vi "SEScontrol.vi"() -> ()   [LabVIEW 2015]
uses:
  <userlib>/caLab/Private/Get_PV-1D.vi
  user32.dll
  <vilib>/picture/picture.llb/imagedata.ctl
panel:
  out "error out":errorcluster
  out "Waveform Chart":u8(graph)
  out "SES:ScreenCount":u8
  out "SES:Screen":picture
  out "SPEAR_STATE_bool":bool
  out "SPEAR_STATE":dbl
  out "SES:BUSY":bool
  out "SES:Stop_REQ":i8
  out "SES:Run_REQ":i8
  out "SES:Cal_OFF_REQ":i8
  out "SES:Cal_On_REQ":i8
  in  "SES:Cal_Off":bool caption="Play"
  in  "SES:Cal_On":bool caption="Play"
  in  "SES:Kin_Energy":dbl=350.0 min=5.0 max=900.0
  in  "exit":bool
  in  "SES:Run":bool caption="Play"
  in  "SES:Stop":bool
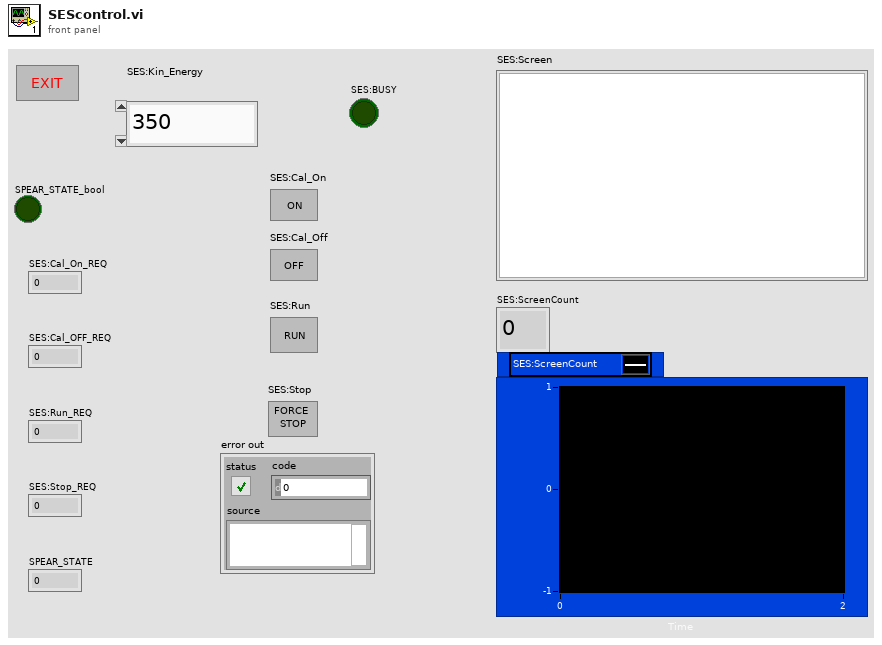
[diagram p1: front panel]
types:
  T1 = typedef "imagedata.ctl" = cluster{"image type":i32, "image depth":i32, "image":u8[], "mask":u8[], "colors":u32[], "Rectangle":cluster{"left":i16, "top":i16, "right":i16, "bottom":i16}}
  T2 = enum16{"Mouse Left", "Mouse Right", "Break", "Mouse Middle", "Backspace", "Tabulator", "FormFeed", "Return", "Shift", "Control", "Alternate", "Pause", "CapsLock", "Escape", "Space", "Page Up", "Page Down", "End", "Home", "Left", "Up", "Right", "Down", "Select", "Print", "Execute", "Snapshot", "Insert", "Delete", "Help", "0", "1", "2", "3", "4", "5", "6", "7", "8", "9", "A", "B", "C", "D", "E", "F", "G", "H", "I", "J", "K", "L", "M", "N", "O", "P", "Q", "R", "S", "T", "U", "V", "W", "X", "Y", "Z", "Win Left", "Win Right", "Context Menu", "Num 0", "Num 1", "Num 2", "Num 3", "Num 4", "Num 5", "Num 6", "Num 7", "Num 8", "Num 9", "Multiply", "Add", "Separator", "Subtract", "Decimal", "Divide", "F1", "F2", "F3", "F4", "F5", "F6", "F7", "F8", "F9", "F10", "F11", "F12", "F13", "F14", "F15", "F16", "F17", "F18", "F19", "F20", "F21", "F22", "F23", "F24", "NumLock", "Scroll", "Shift Left", "Shift Right", "Control Left", "Control Right", "Alternate Left", "Alternate Right", "Attn", "CrSel", "ExSel", "ErEOF", "Play", "Zoom", "Noname", "PA1", "OEM Clear", "Germany <", "Germany ^", "Germany ß", "Germany ´", "Germany ü", "Germany +", "Germany ö", "Germany ä", "Germany #", "Germany ,", "Germany .", "Germany -"}
  T3 = enum16{"NO", "SHIFT", "CTRL", "ALT", "SHIFT + CTRL", "SHIFT + ALT", "CTRL + ALT", "SHIFT + CTRL + ALT"}
  T4 = typedef "LVRectTypeDef.ctl" = cluster{"left":i16, "top":i16, "right":i16, "bottom":i16}
  T5 = typedef "WindowHandle" = refnum<k1>
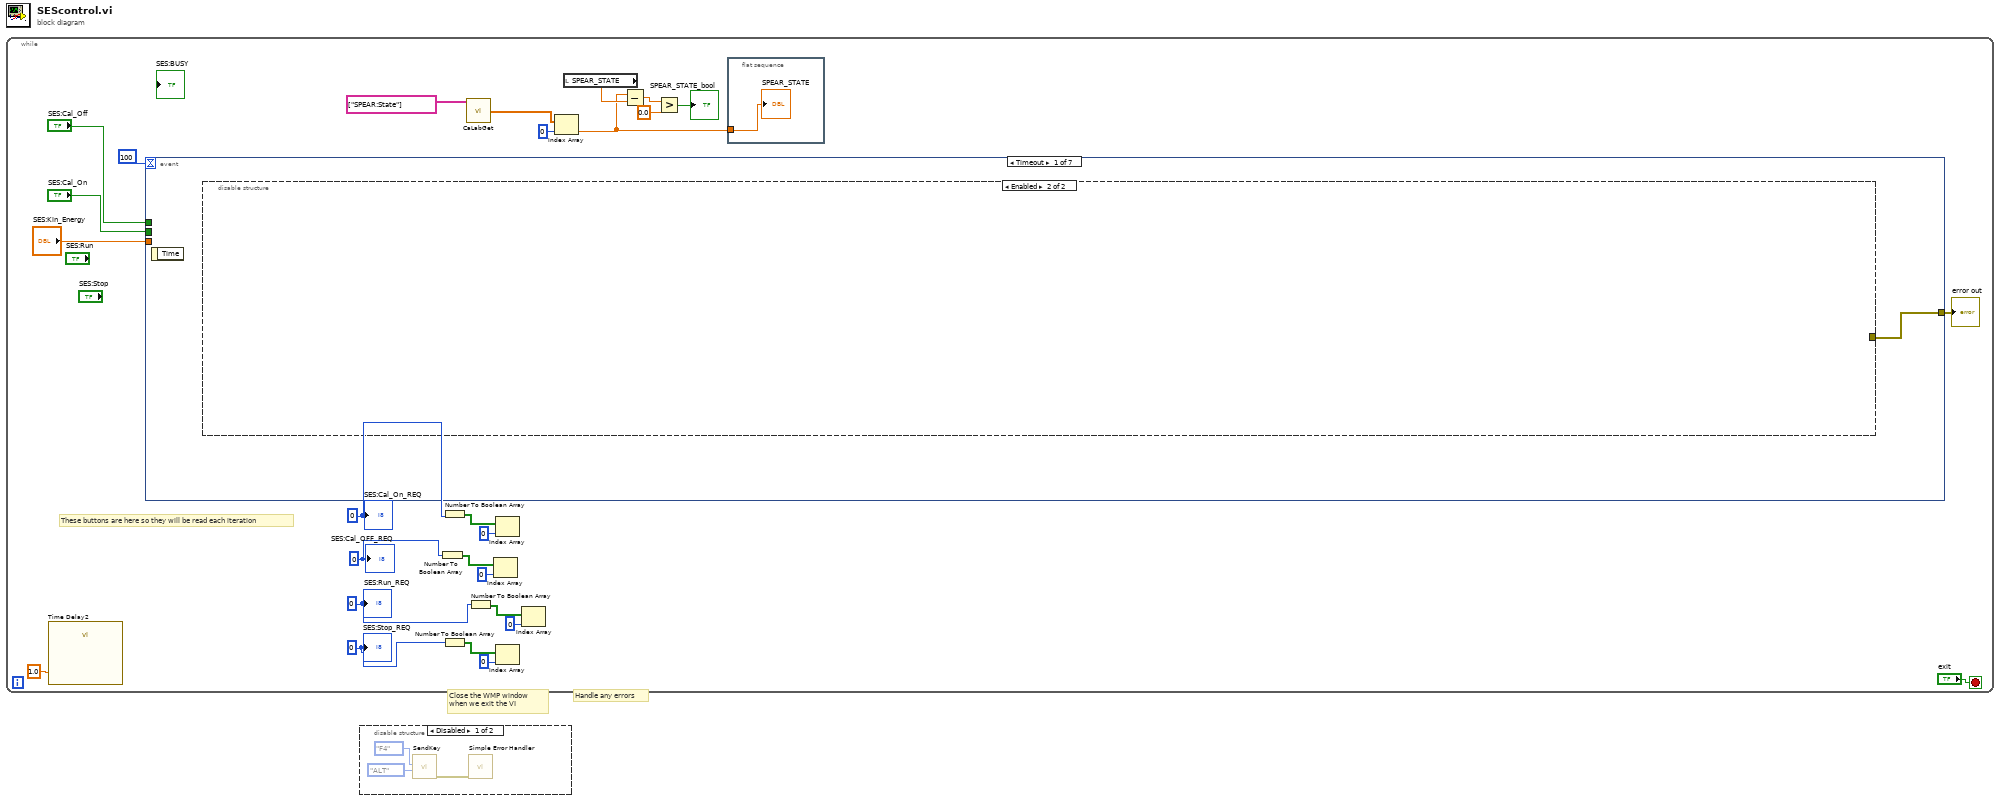
[diagram p0: block diagram]
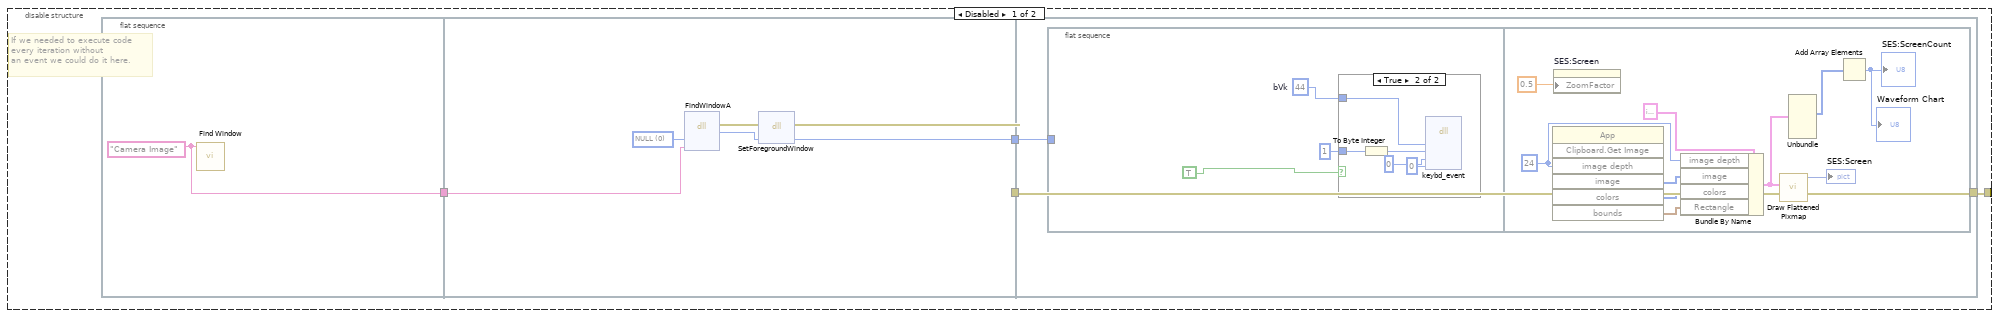
[diagram p3: hidden frame]
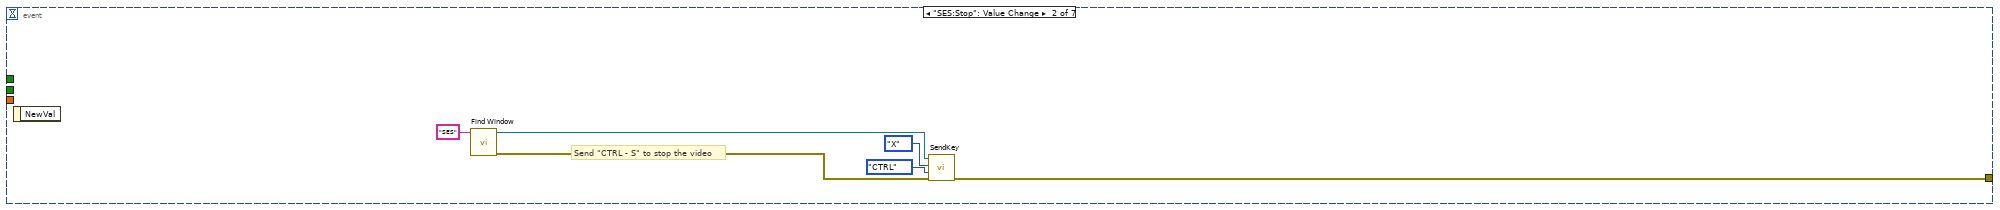
[diagram p5: hidden frame]
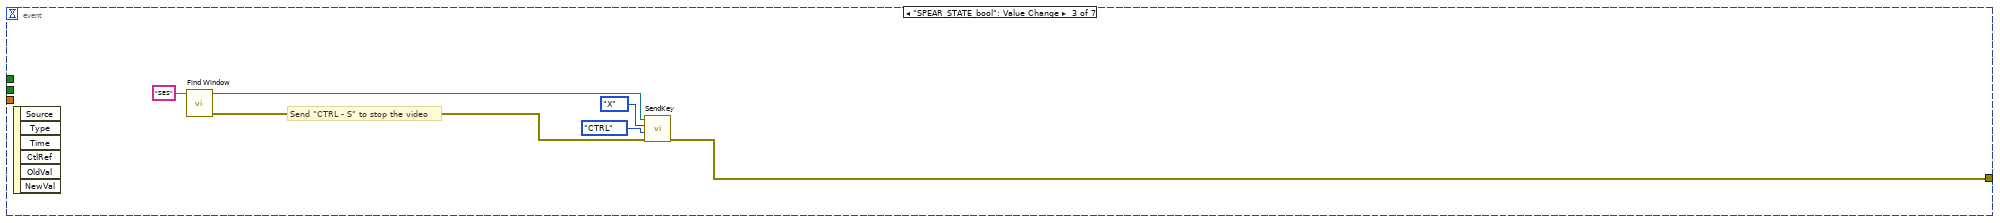
[diagram p6: hidden frame]
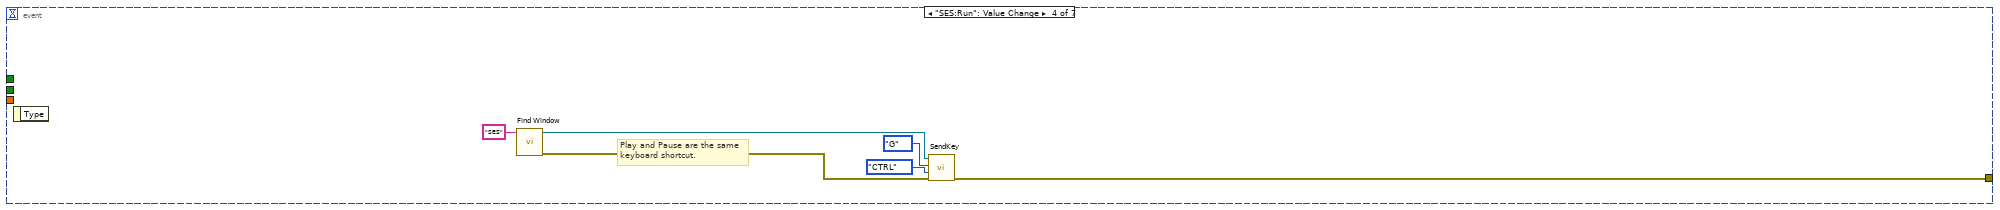
[diagram p7: hidden frame]
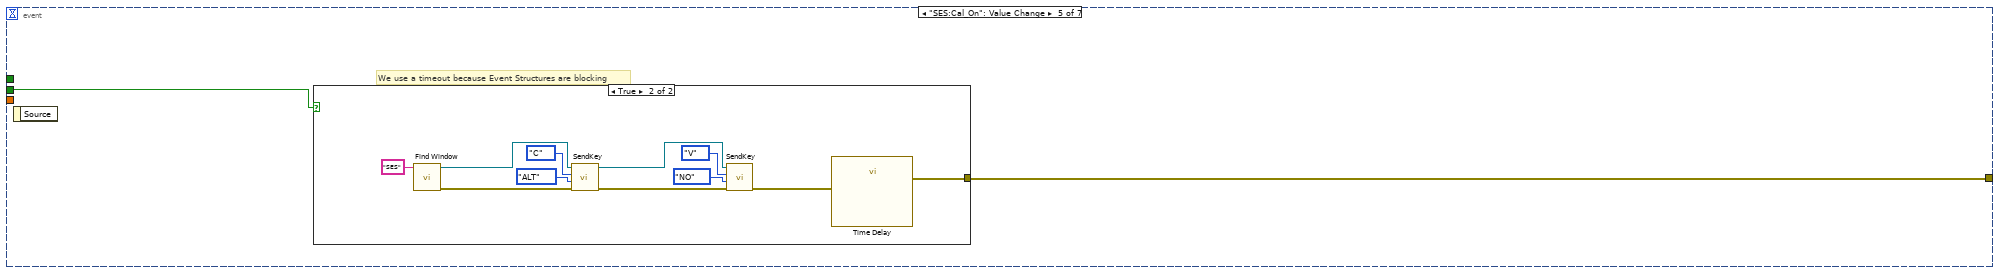
[diagram p8: hidden frame]
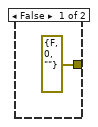
[diagram p9: hidden frame]
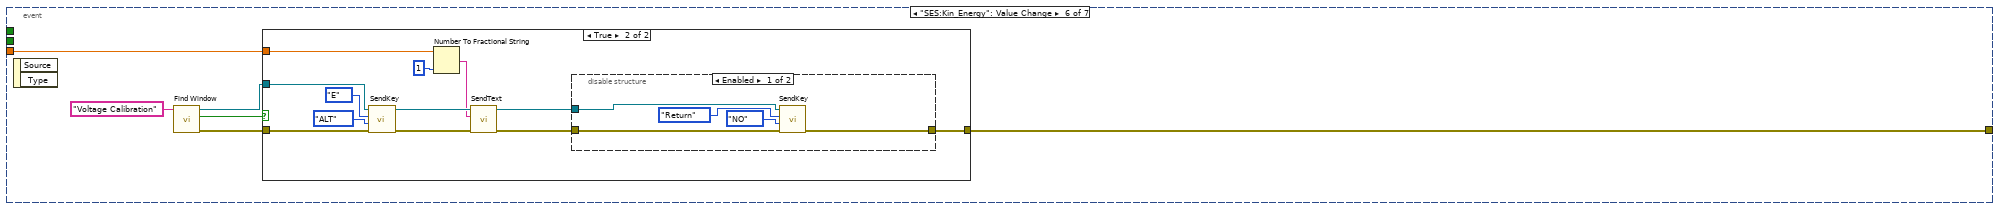
[diagram p10: hidden frame]
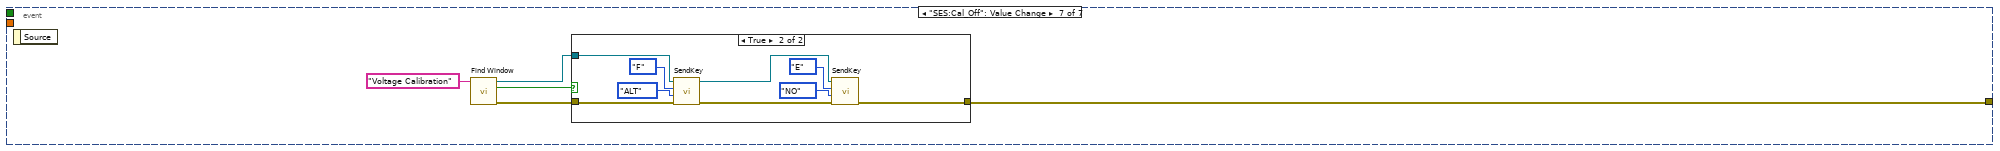
[diagram p13: hidden frame]
diagram:
  # "Handle any errors"
  # "Close the WMP window\nwhen we exit the VI"
  n1 = while {
    stop <- "exit" stop-if-true
    w10 = i8 0 ("SES:Stop_REQ")
    w11 = i8 0 ("SES:Run_REQ")
    w12 = i8 0 ("SES:Cal_Off_REQ")
    w21 = i8 0 ("SES:Cal_On_REQ")
    # "These buttons are here so they will be read each iteration"
    n2 = call "Time Delay2"("Delay Time (s)"=1.0) -> ()  [unwired: 10 in, 1 out]
    n3 = event shown="[0] Timeout" {
      selector: _ -> [_ _ _ _ _ _ _]
      dyn-events: _ -> [_ _ _ _ _ _ _]
      timeout: 100 -> [_ _ _ _ _ _ _]
      tunnel: [w29 w66 w67 w78 w80 w93 w121] -> w1
      tunnel: "SES:Cal_On" -> [_ _ _ _ w79 _ _]
      tunnel: "SES:Cal_Off" -> [_ _ _ _ _ _ _]
      tunnel: "SES:Kin_Energy" -> [_ _ _ _ _ w95 _]
      event Timeout {
        n4 = event-data() -> ()  [unwired: 1 in, 1 out]
        n5 = disable-structure shown="Enabled" {
          disable-tunnel: [w30 _] -> w29
          frame Disabled {
            # "If we needed to execute code\nevery iteration without\nan event we could do it here."
            n6 = flat-sequence {
              tunnel: [w34] -> w33
              tunnel: w33 -> [w37]
              tunnel: [w36] -> w32
              tunnel: [w35] -> w31
              tunnel: [w42] -> w30
              tunnel: w32 -> [w42]
              tunnel: w31 -> [w41]
              frame #0 {
                w34 = "Camera Image" ("WindowName")
                n7 = call "Find Window.vi"("WindowName"=w34) -> ()  [unwired: 8 in, 3 out]
              }
              frame #1 {
                w40 = 0 items=["NULL"]
                n8 = dll-call lib="user32.dll" fn="FindWindowA" label="FindWindow"("lpszClassName"=w40, "lpszWindowName"=w37) -> (error out=w38:errorcluster, "hWnd"=w39:u32)  [unwired: 4 in, 2 out]
                n9 = dll-call lib="user32.dll" fn="SetForegroundWindow"(error in=w38, "Handle"=w39) -> (error out=w36:errorcluster, "Handle"=w35:i32)  [unwired: 2 in, 2 out]
              }
              frame #2 {
                n10 = flat-sequence {
                  tunnel: w41 -> [_]
                  frame #0 {
                    w44 = u32 44  # bVk
                    n11 = case shown="True" TRUE {
                      tunnel: i16 1 -> [_ w48]
                      tunnel: w44 -> [_ w47]
                      frame False {
                      }
                      frame True {
                        n12 = To Byte Integer(number=w48) -> (8bit integer=w50:i8)
                        n13 = dll-call lib="USER32.DLL" fn="keybd_event"(w47, w50, 0 ("Input Value"), 0) -> ()  [unwired: 7 in, 3 out]
                      }
                    }
                  }
                  frame #1 {
                    w60 = 24 ("image depth")
                    n14 = invoke class="App" method="Clipboard.Get Image"("image depth"=w60) -> ("image"=w57:u8[], "colors"=w58:u32[], "bounds"=w59:T4)  [unwired: 6 in, 4 out]
                    n15 = property on="SES:Screen" class="Pict"("ZoomFactor"=sgl 0.5 ("Zoom Factor")) -> ()  [unwired: 2 in, 2 out]
                    n16 = Bundle By Name(cluster=T1 {"image type"=0, "image depth"=0, "image"=[], "mask"=[], "colors"=[], "Rectangle"={"left"=0, "top"=0, "right"=0, "bottom"=0}} ("image data"), "image depth"=w60, "image"=w57, "colors"=w58, "Rectangle"=w59) -> (w53:T1)
                    n17 = call <vilib>:"Draw Flattened Pixmap.vi"("image data"=w53) -> ("new picture"=→"SES:Screen":picture)  [unwired: 1 in, 7 out]
                    n18 = Unbundle(w53) -> ("image"=w52:u8[])  [unwired: 5 out]
                    n19 = Add Array Elements(numeric array=w52) -> (sum=→"SES:ScreenCount" →"Waveform Chart":u8)
                  }
                }
              }
            }
          }
          frame Enabled {
          }
        }
      }
      event "SES:Stop": Value Change {
        # "Send \"CTRL - S\" to stop the video"
        n20 = event-data() -> ()  [unwired: 1 in, 1 out]
        n21 = call "Find Window.vi"("WindowName"="SES") -> ("error out"=w61:errorcluster, "WindowHandle"=w62:T5)  [unwired: 8 in, 1 out]
        n22 = call "SendKey.vi"("error in (no error)"=w61, "ShiftState"=T3."CTRL", "Virtual Key"=T2."X", "WindowHandle"=w62) -> ("error out"=w66:errorcluster)  [unwired: 2 in, 1 out]
      }
      event "SPEAR_STATE_bool": Value Change {
        # "Send \"CTRL - S\" to stop the video"
        n23 = event-data() -> ()  [unwired: 1 in, 6 out]
        n24 = call "Find Window.vi"("WindowName"="SES") -> ("error out"=w68:errorcluster, "WindowHandle"=w69:T5)  [unwired: 8 in, 1 out]
        n25 = call "SendKey.vi"("error in (no error)"=w68, "ShiftState"=T3."CTRL", "Virtual Key"=T2."X", "WindowHandle"=w69) -> ("error out"=w67:errorcluster)  [unwired: 2 in, 1 out]
      }
      event "SES:Run": Value Change {
        # "Play and Pause are the same\nkeyboard shortcut."
        n26 = event-data() -> ()  [unwired: 1 in, 1 out]
        n27 = call "Find Window.vi"("WindowName"="SES") -> ("error out"=w73:errorcluster, "WindowHandle"=w74:T5)  [unwired: 8 in, 1 out]
        n28 = call "SendKey.vi"("error in (no error)"=w73, "ShiftState"=T3."CTRL", "Virtual Key"=T2."G", "WindowHandle"=w74) -> ("error out"=w78:errorcluster)  [unwired: 2 in, 1 out]
      }
      event "SES:Cal_On": Value Change {
        # "We use a timeout because Event Structures are blocking"
        n29 = event-data() -> ()  [unwired: 1 in, 1 out]
        n30 = case shown="True" w79 {
          tunnel: [errorcluster {"status"=FALSE, "code"=0, "source"=""} ("error out") w82] -> w80
          frame False {
          }
          frame True {
            n31 = call "Find Window.vi"("WindowName"="SES") -> ("error out"=w83:errorcluster, "WindowHandle"=w84:T5)  [unwired: 8 in, 1 out]
            n32 = call "SendKey.vi"("error in (no error)"=w83, "ShiftState"=T3."ALT", "Virtual Key"=T2."C", "WindowHandle"=w84) -> ("error out"=w89:errorcluster, "Previous WindowHandle"=w88:T5)  [unwired: 2 in]
            n33 = call "SendKey.vi"("error in (no error)"=w89, "ShiftState"=T3."NO", "Virtual Key"=T2."V", "WindowHandle"=w88) -> ("error out"=w86:errorcluster)  [unwired: 2 in, 1 out]
            n34 = call "Time Delay"("error in (no error)"=w86) -> ("error out"=w82:errorcluster)  [unwired: 10 in]
          }
        }
      }
      event "SES:Kin_Energy": Value Change {
        n35 = event-data() -> ()  [unwired: 1 in, 2 out]
        n36 = call "Find Window.vi"("WindowName"="Voltage Calibration") -> ("error out"=w97:errorcluster, "WindowFound"=w96:bool, "WindowHandle"=w98:T5)  [unwired: 8 in]
        n37 = case shown="True" w96 {
          tunnel: w98 -> [_ w111]
          tunnel: w97 -> [w99 w108]
          tunnel: [w99 w103] -> w93
          tunnel: w95 -> [_ w100]
          frame False {
          }
          frame True {
            n38 = call "SendKey.vi"("error in (no error)"=w108, "ShiftState"=T3."ALT", "Virtual Key"=T2."E", "WindowHandle"=w111) -> ("error out"=w106:errorcluster, "Previous WindowHandle"=w107:T5)  [unwired: 2 in]
            n39 = Number To Fractional String(number=w100, precision (6)=i16 1) -> (F-format string=w101:string)  [unwired: 2 in]
            n40 = call "SendText.vi"("error in (no error)"=w106, "Text"=w101, "WindowHandle"=w107) -> ("error out"=w104:errorcluster, "Previous WindowHandle"=w105:T5)  [unwired: 3 in]
            n41 = disable-structure shown="Enabled" {
              disable-tunnel: w105 -> [w116 _]
              disable-tunnel: w104 -> [w113 _]
              disable-tunnel: [w112 _] -> w103
              frame Enabled {
                n42 = call "SendKey.vi"("error in (no error)"=w113, "ShiftState"=T3."NO", "Virtual Key"=T2."Return", "WindowHandle"=w116) -> ("error out"=w112:errorcluster)  [unwired: 2 in, 1 out]
              }
              frame Disabled {
              }
            }
          }
        }
      }
      event "SES:Cal_Off": Value Change {
        n43 = event-data() -> ()  [unwired: 1 in, 1 out]
        n44 = call "Find Window.vi"("WindowName"="Voltage Calibration") -> ("error out"=w118:errorcluster, "WindowFound"=w117:bool, "WindowHandle"=w119:T5)  [unwired: 8 in]
        n45 = case shown="True" w117 {
          tunnel: w119 -> [_ w131]
          tunnel: w118 -> [w122 w128]
          tunnel: [w122 w123] -> w121
          frame False {
          }
          frame True {
            n46 = call "SendKey.vi"("error in (no error)"=w128, "ShiftState"=T3."ALT", "Virtual Key"=T2."F", "WindowHandle"=w131) -> ("error out"=w124:errorcluster, "Previous WindowHandle"=w125:T5)  [unwired: 2 in]
            n47 = call "SendKey.vi"("error in (no error)"=w124, "ShiftState"=T3."NO", "Virtual Key"=T2."E", "WindowHandle"=w125) -> ("error out"=w123:errorcluster)  [unwired: 2 in, 1 out]
          }
        }
      }
    }
    "error out" <- w1
    n48 = Number To Boolean Array(number=w12) -> (Boolean array=w18:bool[])
    n49 = Number To Boolean Array(number=w21) -> (Boolean array=w20:bool[])
    n50 = Number To Boolean Array(number=w10) -> (Boolean array=w14:bool[])
    n51 = call-poly <userlib>:"CaLabGet.vi"("PV Names"=string[] ["SPEAR:State"]) -> ("1rst Value (number)"=w8:dbl[])  [unwired: 8 in, 6 out]
    n52 = Number To Boolean Array(number=w11) -> (Boolean array=w16:bool[])
    n53 = Index Array(array=w18, index=0) -> ()  [unwired: 1 out]
    n54 = Index Array(array=w20, index=0) -> ()  [unwired: 1 out]
    n55 = Index Array(array=w14, index=0) -> ()  [unwired: 1 out]
    n56 = Index Array(array=w16, index=0) -> ()  [unwired: 1 out]
    n57 = Index Array(array=w8, index=0) -> (element=w2:dbl)
    n58 = local read "SPEAR_STATE"() -> (w6:dbl)
    n59 = Subtract(x=w2, y=w6) -> (x-y=w5:dbl)
    n60 = Greater?(x=w5, y=0.0) -> (0:→"SPEAR_STATE_bool":bool)
    n61 = flat-sequence {
      tunnel: w2 -> [w28]
      frame #0 {
        "SPEAR_STATE" <- w28
      }
    }
    "SES:Cal_On_REQ" <- w21
    "SES:Cal_OFF_REQ" <- w12
    "SES:Run_REQ" <- w11
    "SES:Stop_REQ" <- w10
  }
  n62 = disable-structure shown="Disabled" {
    frame Disabled {
      n63 = call "SendKey.vi"("ShiftState"=T3."ALT", "Virtual Key"=T2."F4") -> ("error out"=w132:errorcluster)  [unwired: 4 in, 1 out]
      n64 = call <vilib>:"Simple Error Handler.vi"("error in (no error)"=w132) -> ()  [unwired: 4 in, 5 out]
    }
    frame Enabled {
    }
  }
